vi "Convert2ValidCylinderCalibrParams.vi"(1 "CylinderCalibrNew in":T1) -> (0 "CylinderCalibrNew out":T1)   [LabVIEW 2017]
uses:
  CylinderCalibrNew.ctl
  Initialization.lvlib
panel:
  # "Convert the calibration to effective values"
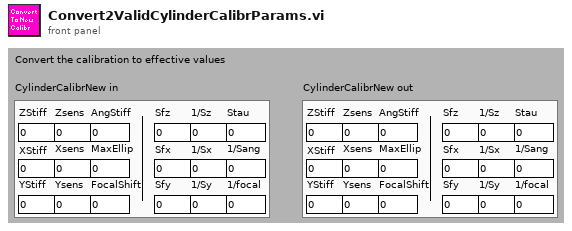
[diagram p1: front panel]
types:
  T1 = typedef "Initialization.lvlib/CylinderCalibrNew.ctl" = cluster{"ZStiff":dbl, "Zsens":dbl, "AngStiff":dbl, "XStiff":dbl, "Xsens":dbl, "MaxEllip":dbl, "YStiff":dbl, "Ysens":dbl, "FocalShift":dbl, "Sfz":dbl, "1/Sz":dbl, "Stau":dbl, "Sfx":dbl, "1/Sx":dbl, "1/Sang":dbl, "Sfy":dbl, "1/Sy":dbl, "1/focal":dbl}
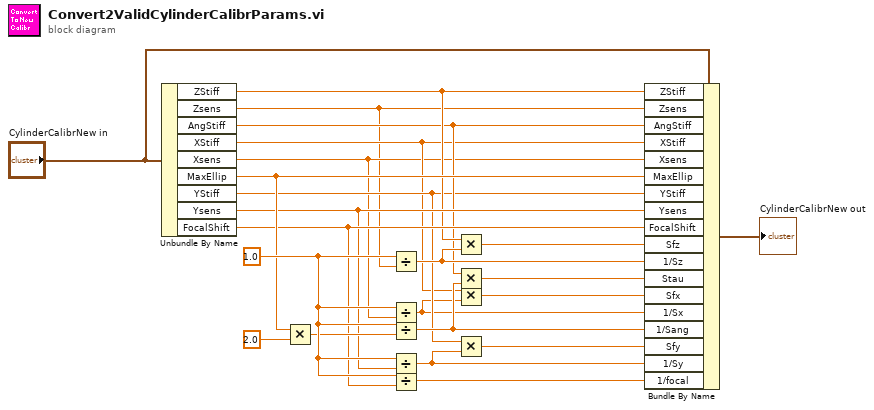
[diagram p0: block diagram]
diagram:
  w21 = 1.0 ("x")
  n1 = Unbundle By Name("CylinderCalibrNew in") -> ("ZStiff"=w13:dbl, "Zsens"=w1:dbl, "AngStiff"=w10:dbl, "XStiff"=w4:dbl, "Xsens"=w2:dbl, "MaxEllip"=w19:dbl, "YStiff"=w7:dbl, "Ysens"=w16:dbl, "FocalShift"=w17:dbl)
  n2 = Multiply(x=w19, y=2.0 ("x")) -> (x*y=w20:dbl)
  n3 = Divide(x=w21, y=w1) -> (x/y=w14:dbl)
  n4 = Divide(x=w21, y=w2) -> (x/y=w5:dbl)
  n5 = Divide(x=w21, y=w20) -> (x/y=w11:dbl)
  n6 = Divide(x=w21, y=w16) -> (x/y=w8:dbl)
  n7 = Divide(x=w21, y=w17) -> (x/y=w18:dbl)
  n8 = Multiply(x=w13, y=w14) -> (x*y=w15:dbl)
  n9 = Multiply(x=w10, y=w11) -> (x*y=w12:dbl)
  n10 = Multiply(x=w4, y=w5) -> (x*y=w6:dbl)
  n11 = Multiply(x=w7, y=w8) -> (x*y=w9:dbl)
  n12 = Bundle By Name(cluster="CylinderCalibrNew in", "ZStiff"=w13, "Zsens"=w1, "AngStiff"=w10, "XStiff"=w4, "Xsens"=w2, "MaxEllip"=w19, "YStiff"=w7, "Ysens"=w16, "FocalShift"=w17, "Sfz"=w15, "1/Sz"=w14, "Stau"=w12, "Sfx"=w6, "1/Sx"=w5, "1/Sang"=w11, "Sfy"=w9, "1/Sy"=w8, "1/focal"=w18) -> (→"CylinderCalibrNew out":T1)
